vi "LVH5Pget_default.vi"(6 "error in (no error)":errorcluster) -> (0 "error out":errorcluster, 3 "HDF5 Property List Ref":T2)   [LabVIEW 2017]
doc: "Gets the default property list for the specified property class"
uses:
  <vilib>/UPVI/lvhdf5/library.llb/HDF5 Ref.ctl
  <vilib>/UPVI/lvhdf5/property.llb/LVH5PClassId.ctl
panel:
  in  "Property List Class":T1=enum."H5P_FILE_CREATE"
  # "LVHDF5 Toolkit\nCopyright (c) 2005-2013 by Jason D. Sommerville\nCopyright (c) 2014 by UPVI, LLC.\n\nThis use and distribution of this file is governed by the terms found in \nLICENSE.txt distributed with this toolkit and installed at\n <user.lib>\\_lvhdf5\\LICENSE.txt"
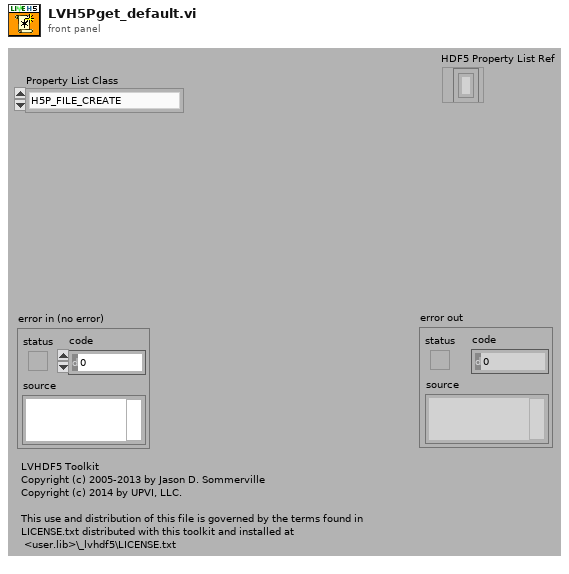
[diagram p1: front panel]
types:
  T1 = typedef "LVH5PClassId.ctl" = enum32{"H5P_ROOT", "H5P_OBJECT_CREATE", "H5P_FILE_CREATE", "H5P_FILE_ACCESS", "H5P_DATASET_CREATE", "H5P_DATASET_ACCESS", "H5P_DATASET_XFER", "H5P_FILE_MOUNT", "H5P_GROUP_CREATE", "H5P_GROUP_ACCESS", "H5P_DATATYPE_CREATE", "H5P_DATATYPE_ACCESS", "H5P_STRING_CREATE", "H5P_ATTRIBUTE_CREATE", "H5P_OBJECT_COPY", "H5P_LINK_CREATE", "H5P_LINK_ACCESS"}
  T2 = typedef "HDF5 Ref.ctl" = refnum<k1>
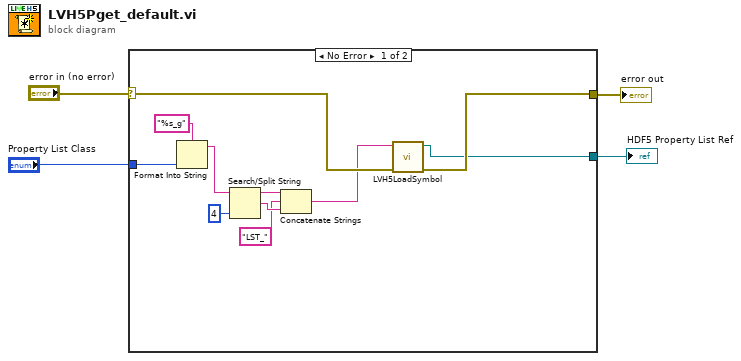
[diagram p0: block diagram]
diagram:
  n1 = case shown="No Error" "error in (no error)" {
    selector: "error in (no error)" -> [w13 w16]
    tunnel: [w12 w16] -> w3
    tunnel: "Property List Class" -> [w14 _]
    tunnel: [w11 _] -> w2
    frame No Error {
      n2 = Format Into String(format string="%s_g", w14) -> (resulting string=w6:string)  [unwired: 2 in, 1 out]
      n3 = Search/Split String(string=w6, offset (0)=4) -> (substring before match=w9:string, match + rest of string=w8:string)  [unwired: 1 in, 1 out]
      n4 = Concatenate Strings(w9, "LST_" ("string"), w8) -> (w5:string)
      n5 = call <vilib>:"LVH5LoadSymbol.vi"("error in (no error)"=w13, "Symbol"=w5) -> ("error out"=w12:errorcluster, "Refnum out"=w11:T2)  [unwired: 8 in]
    }
    frame Error {
    }
  }
  "error out" <- w3
  "HDF5 Property List Ref" <- w2
